vi "RecordSA.vi"() -> ()   [LabVIEW 2020]
uses:
  <vilib>/Utility/file.llb/Write Delimited Spreadsheet (DBL).vi
panel:
  out "sa":dbl[](graph)
  out "size(s)":i32
  out "SA1":dbl[](array[numeric])
  in  "Stop?":bool
  out "error out":errorcluster
  in  "SA":refnum<visa-resource-name>="TCPIP::192.168.100.230::inst0::INSTR"
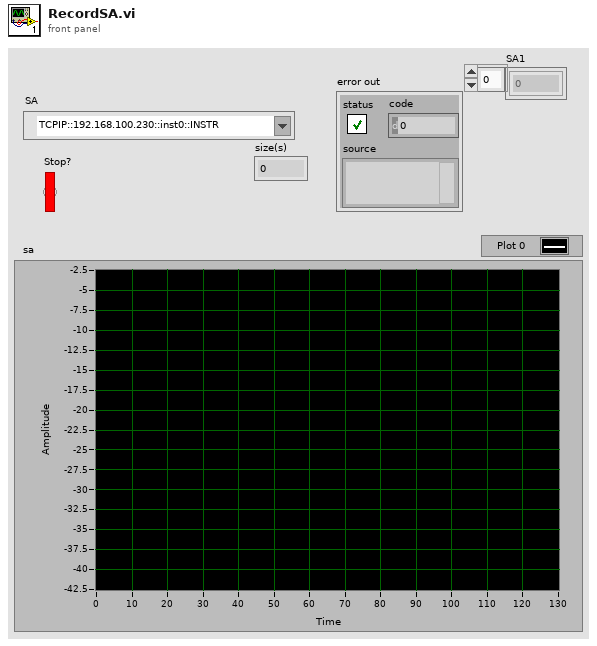
[diagram p1: front panel]
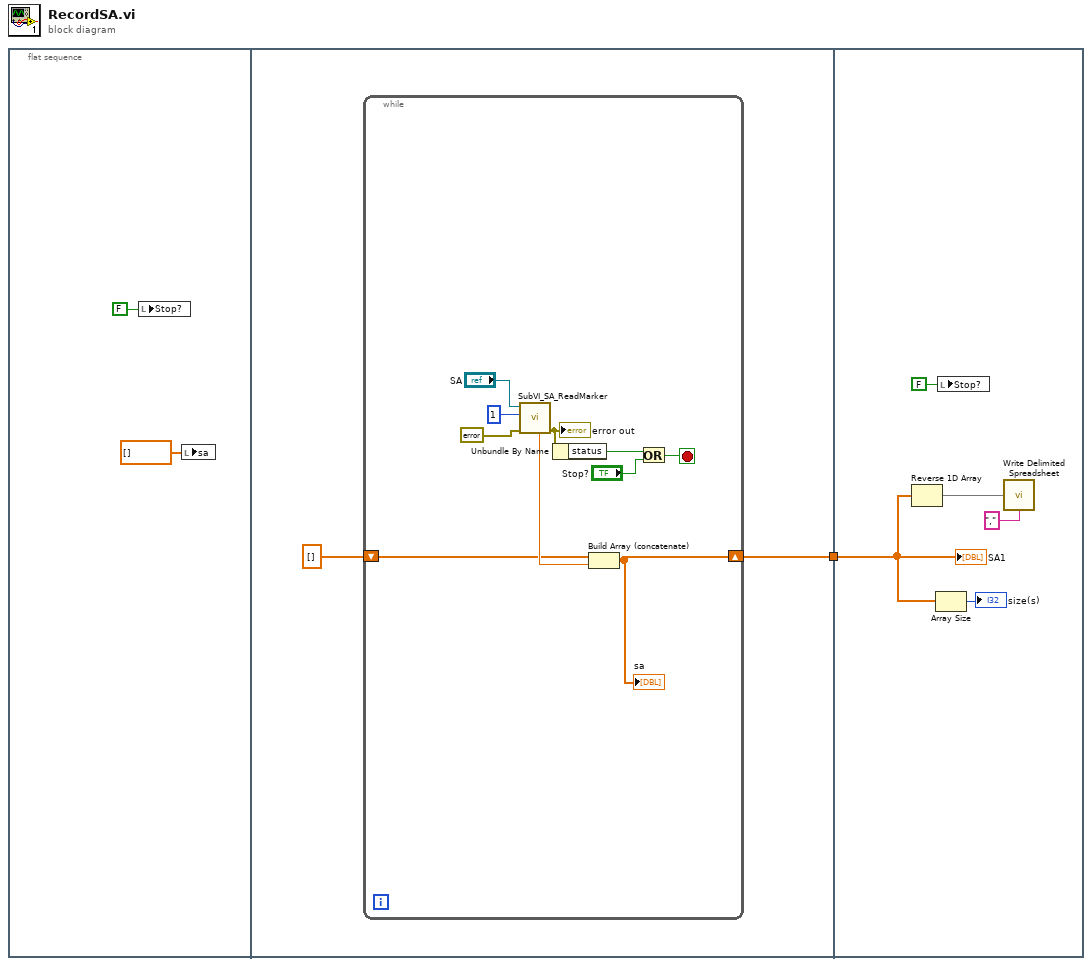
[diagram p0: block diagram]
diagram:
  n1 = flat-sequence {
    tunnel: [w4] -> w1
    tunnel: w1 -> [w17]
    frame #0 {
      n2 = local write "Stop?"(FALSE ("Stop?")) -> ()
      n3 = local write "sa"(dbl[] [] ("sa")) -> ()
    }
    frame #1 {
      n4 = while {
        shift-right: [w6] -> w4
        shift-left: dbl[] [] ("SA1") -> [w7]
        stop <- w9 stop-if-true
        n5 = call "SubVI_SA_ReadMarker.vi"("error in (no error)"=errorcluster {"status"=FALSE, "code"=0, "source"=""}, "AvgTimes"=1, "VISA resource name"="SA") -> ("error out"=w12:errorcluster, "Marker Power"=w8:dbl)  [unwired: 5 in, 2 out]
        "error out" <- w12
        n6 = Unbundle By Name(w12) -> ("status"=w11:bool)
        n7 = Build Array (concatenate)(w7, w8) -> (w6:dbl[])
        "sa" <- w6
        n8 = Or(x=w11, y="Stop?") -> (x .or. y?=w9:bool)
      }
    }
    frame #2 {
      n9 = Reverse 1D Array(array=w17) -> (reversed array=w16:dbl[])
      n10 = Array Size(array=w17) -> (size(s)=→"size(s)":i32)
      n11 = local write "Stop?"(FALSE ("Stop?")) -> ()
      n12 = call-poly <vilib>:"Write Delimited Spreadsheet.vi"("1D data"=w16, "delimiter (\\t)"="," ("delimiter (\\t)")) -> ()  [unwired: 12 in, 2 out]
      "SA1" <- w17
    }
  }
